vi "create new function.vi"(11 "function name":string) -> (3 "processing function":T1)   [LabVIEW 2013, in "Logic Sequencer configuration.lvclass"]
uses:
  Logic Sequencer configuration.lvclass
  processing channels.ctl
  <vilib>/NI/Tag Bus Module Framework/channel/TBM channel.lvclass
  <vilib>/NI/Tag Bus Module Framework/channel/channel classification.ctl
  <vilib>/NI/Tag Bus/tag/Data Type.ctl
  <vilib>/NI/Tag Bus/tag/tag descriptor.lvclass
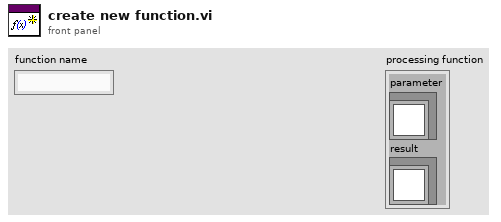
[diagram p1: front panel]
types:
  T1 = typedef "Logic Sequencer configuration.lvclass/processing channels.ctl" = cluster{"parameter":refnum<class "TBM channel.lvclass">, "result":refnum<class "TBM channel.lvclass">}
  T2 = typedef "tag bus.lvlib/tag descriptor.lvclass/Data Type.ctl" = enum16{"Double", "Single", "I64", "I32", "I16", "I8", "U64", "U32", "U16", "U8", "Boolean", "String", "Array of Double", "Array of Single", "Array of I64", "Array of I32", "Array of I16", "Array of I8", "Array of U64", "Array of U32", "Array of U16", "Array of U8", "Array of Boolean", "Array of String"}
  T3 = typedef "TBM channel.lvclass/channel classification.ctl" = enum16{"input data", "output data", "processing parameter", "processing result"}
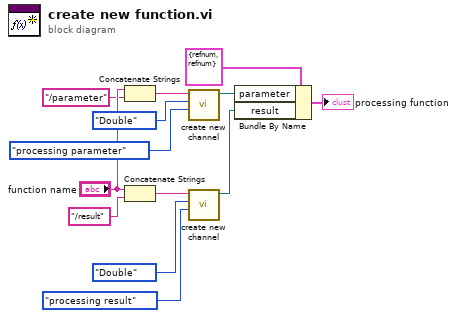
[diagram p0: block diagram]
diagram:
  n1 = Concatenate Strings("function name", "/parameter" ("string")) -> (w4:string)
  n2 = Concatenate Strings("function name", "/result" ("string")) -> (w3:string)
  n3 = call <vilib>:"create new channel.vi"("channel classification"=channel_classification."processing parameter", "data type"=Data_Type."Double", "channel name"=w4) -> ("channel"=w7:refnum<class "TBM channel.lvclass">)  [unwired: 8 in]
  n4 = call <vilib>:"create new channel.vi"("channel classification"=channel_classification."processing result", "data type"=Data_Type."Double", "channel name"=w3) -> ("channel"=w6:refnum<class "TBM channel.lvclass">)  [unwired: 8 in]
  n5 = Bundle By Name(cluster=T1 {"parameter"=refnum, "result"=refnum} ("processing function"), "parameter"=w7, "result"=w6) -> (→"processing function":T1)
